vi "Camera_Crop_X_Axis_2.0.vi"(9 "Detect Movement":bool, 10 "Camera":T5, 11 "Data":T1={"Camera 1"={"Camera1"="", "Cam 1"=FALSE, "CAM1 Model"=enum."a2A5328-15ucBAS", "Cam1 ID"=0}, "Camera 2"={"Camera2"="", "Cam 2"=FALSE, "CAM2 Model"=enum."a2A5328-15ucBAS", "Cam2 ID"=0}, "Image"={"Camera1_Img"=refnum, "Camera2_Img"=refnum, "Img1_Orig_Disp"=refnum, "Img2_Orig_Disp"=refnum, "Img1_Orig_RGB"=refnum, "Img2_Orig_RGB"=refnum, "Blue_Plane_Extract"=refnum, "Subtracted_Plane"=refnum, "Img1_Binary"=refnum, "Img2_Binary"=refnum, "Crop_Mask"=refnum, "Img1_Save"=refnum, "Img2_Save"=refnum, "Img1_Cali_Full"=refnum, "Img2_Cali_Full"=refnum, "Img1_Cali_Detect"=refnum, "Img2_Cali_Detect"=refnum}, "Ques"={"Cam 1 queue"=refnum, "Cam 2 queue"=refnum, "Cam 1 - save queue"=refnum, "Cam 2 - save queue"=refnum, "Image Process Queue Size"=500, "Image Save Queue Size"=500, "Overload threshold"=500, "Max large object threshold"=0}, "Arduino SRS"={"Pinch-valve"="", "Actuator"=FALSE, "Open(T)/Close(F)"=FALSE, "Arduino Uno"=""}, "Pump"={"Port"="", "Connection"=FALSE, "Flush Size"=0, "Command"="", "Pump Size"=enum."None", "Pump"="", "Ready"=FALSE}, "Camera settings"={"Detection settings"={"Sample size threshold"=500, "Detection Region %"=30.0, "Timeout Sample"=200}, "Lens/camera settings"={"Aperture"=enum."Item 0", "Legacy Cam Attributes"=FALSE, "Max Framerate"=100, "Exposure Time"=1000.0, "Framerate"=15}, "Crop settings"={"Cam1"={"Rectangle 1"={"Left"=0, "Top"=0, "Right"=0, "Bottom"=0, "Rotation"=0.0}, "Camera Orientation 1"="", "Pixel to mm 1"=0.0}, "Cam2"={"Rectangle 2"={"Left"=0, "Top"=0, "Right"=0, "Bottom"=0, "Rotation"=0.0}, "Camera Orientation 2"="", "Pixel to mm 2"=0.0}}}, "Arduino ISS"={"Mega F3"="", "Phase3"=FALSE, "Barcode"="", "Sorting sys."=FALSE, "Initial size"=0.0, "Size Interval"=0.0, "Mun. of containers"=0.0, "Container nr."=0.0, "Arduino Mega"=""}, "Img_Capt"=FALSE, "Empty_Refill"=FALSE, "I don't think is in use"={"Light intensity"=100}, "Extended setup"={"Location"="Station", "Latitude"="Station", "Longitude"="Station", "Determiner"="Station", "Sex"="Station", "Station"="", "Collection date"=""}, "Main interface"={"Sample Name"="Test Sample", "Operator"="JFR", "Species Name"="", "Other Notes"=""}, "Tap1"=0, "SystemVersion"=0, "System Serial"="", "Exit"=FALSE, "Kuvette Full"=FALSE, "Core JKI"={"Current VI Reference"=refnum, "Close Panel on Exit?"=FALSE}, "Calibration"={"Calibration 1"=path "C:/Users/au540322/Desktop/IHS_Project/images/Debris/Debris_0/Debris_0_2019_06_01-23-32-49-686.PNG", "Calibration 2"=path "C:/Users/au540322/Desktop/IHS_Project/images/Debris/Debris_0/Debris_0_2019_06_01-23-32-49-686.PNG", "Detect 1"=path "C:/Users/au540322/Desktop/IHS_Project/images/Debris/Debris_0/Debris_0_2019_06_01-23-32-49-686.PNG", "Detect 2"=path "C:/Users/au540322/Desktop/IHS_Project/images/Debris/Debris_0/Debris_0_2019_06_01-23-32-49-686.PNG"}, "Auto Flush"=FALSE} {"SystemVersion" items=["Standard", "XL"]; "Tap1" items=["Session Data", "Extended Setup", "Buffer", "Camera", "Dispenser", "Stats", "Connections"]; "I don't think is in use"."Light intensity" scale=0.0..100.0; "Camera settings"."Crop settings"."Cam2"."Rectangle 2"."Rotation" format="%.2f"; "Camera settings"."Crop settings"."Cam2"."Rectangle 2"."Left" scale=0.0..1024.0; "Camera settings"."Crop settings"."Cam2"."Rectangle 2"."Right" scale=0.0..1024.0; "Camera settings"."Crop settings"."Cam1"."Rectangle 1"."Rotation" format="%.2f"; "Camera settings"."Crop settings"."Cam1"."Rectangle 1"."Left" scale=0.0..1024.0; "Camera settings"."Crop settings"."Cam1"."Rectangle 1"."Right" scale=0.0..1024.0; "Camera settings"."Lens/camera settings"."Framerate" min=1; "Camera settings"."Lens/camera settings"."Max Framerate" min=1; "Camera settings"."Detection settings"."Sample size threshold" min=1; "Pump"."Flush Size" min=0 max=6000 step=100; "Ques"."Overload threshold" min=1; "Ques"."Image Save Queue Size" min=1; "Ques"."Image Process Queue Size" min=1}) -> (1 "Width":i64, 3 "OffsetX":i64)   [LabVIEW 2024]
uses:
  Camera_ID.ctl
  controls/Data_JKI.ctl
  <vilib>/userDefined/High Color/IMAQdx.ctl
  <vilib>/vision/Image Controls.llb/IMAQ Image.ctl
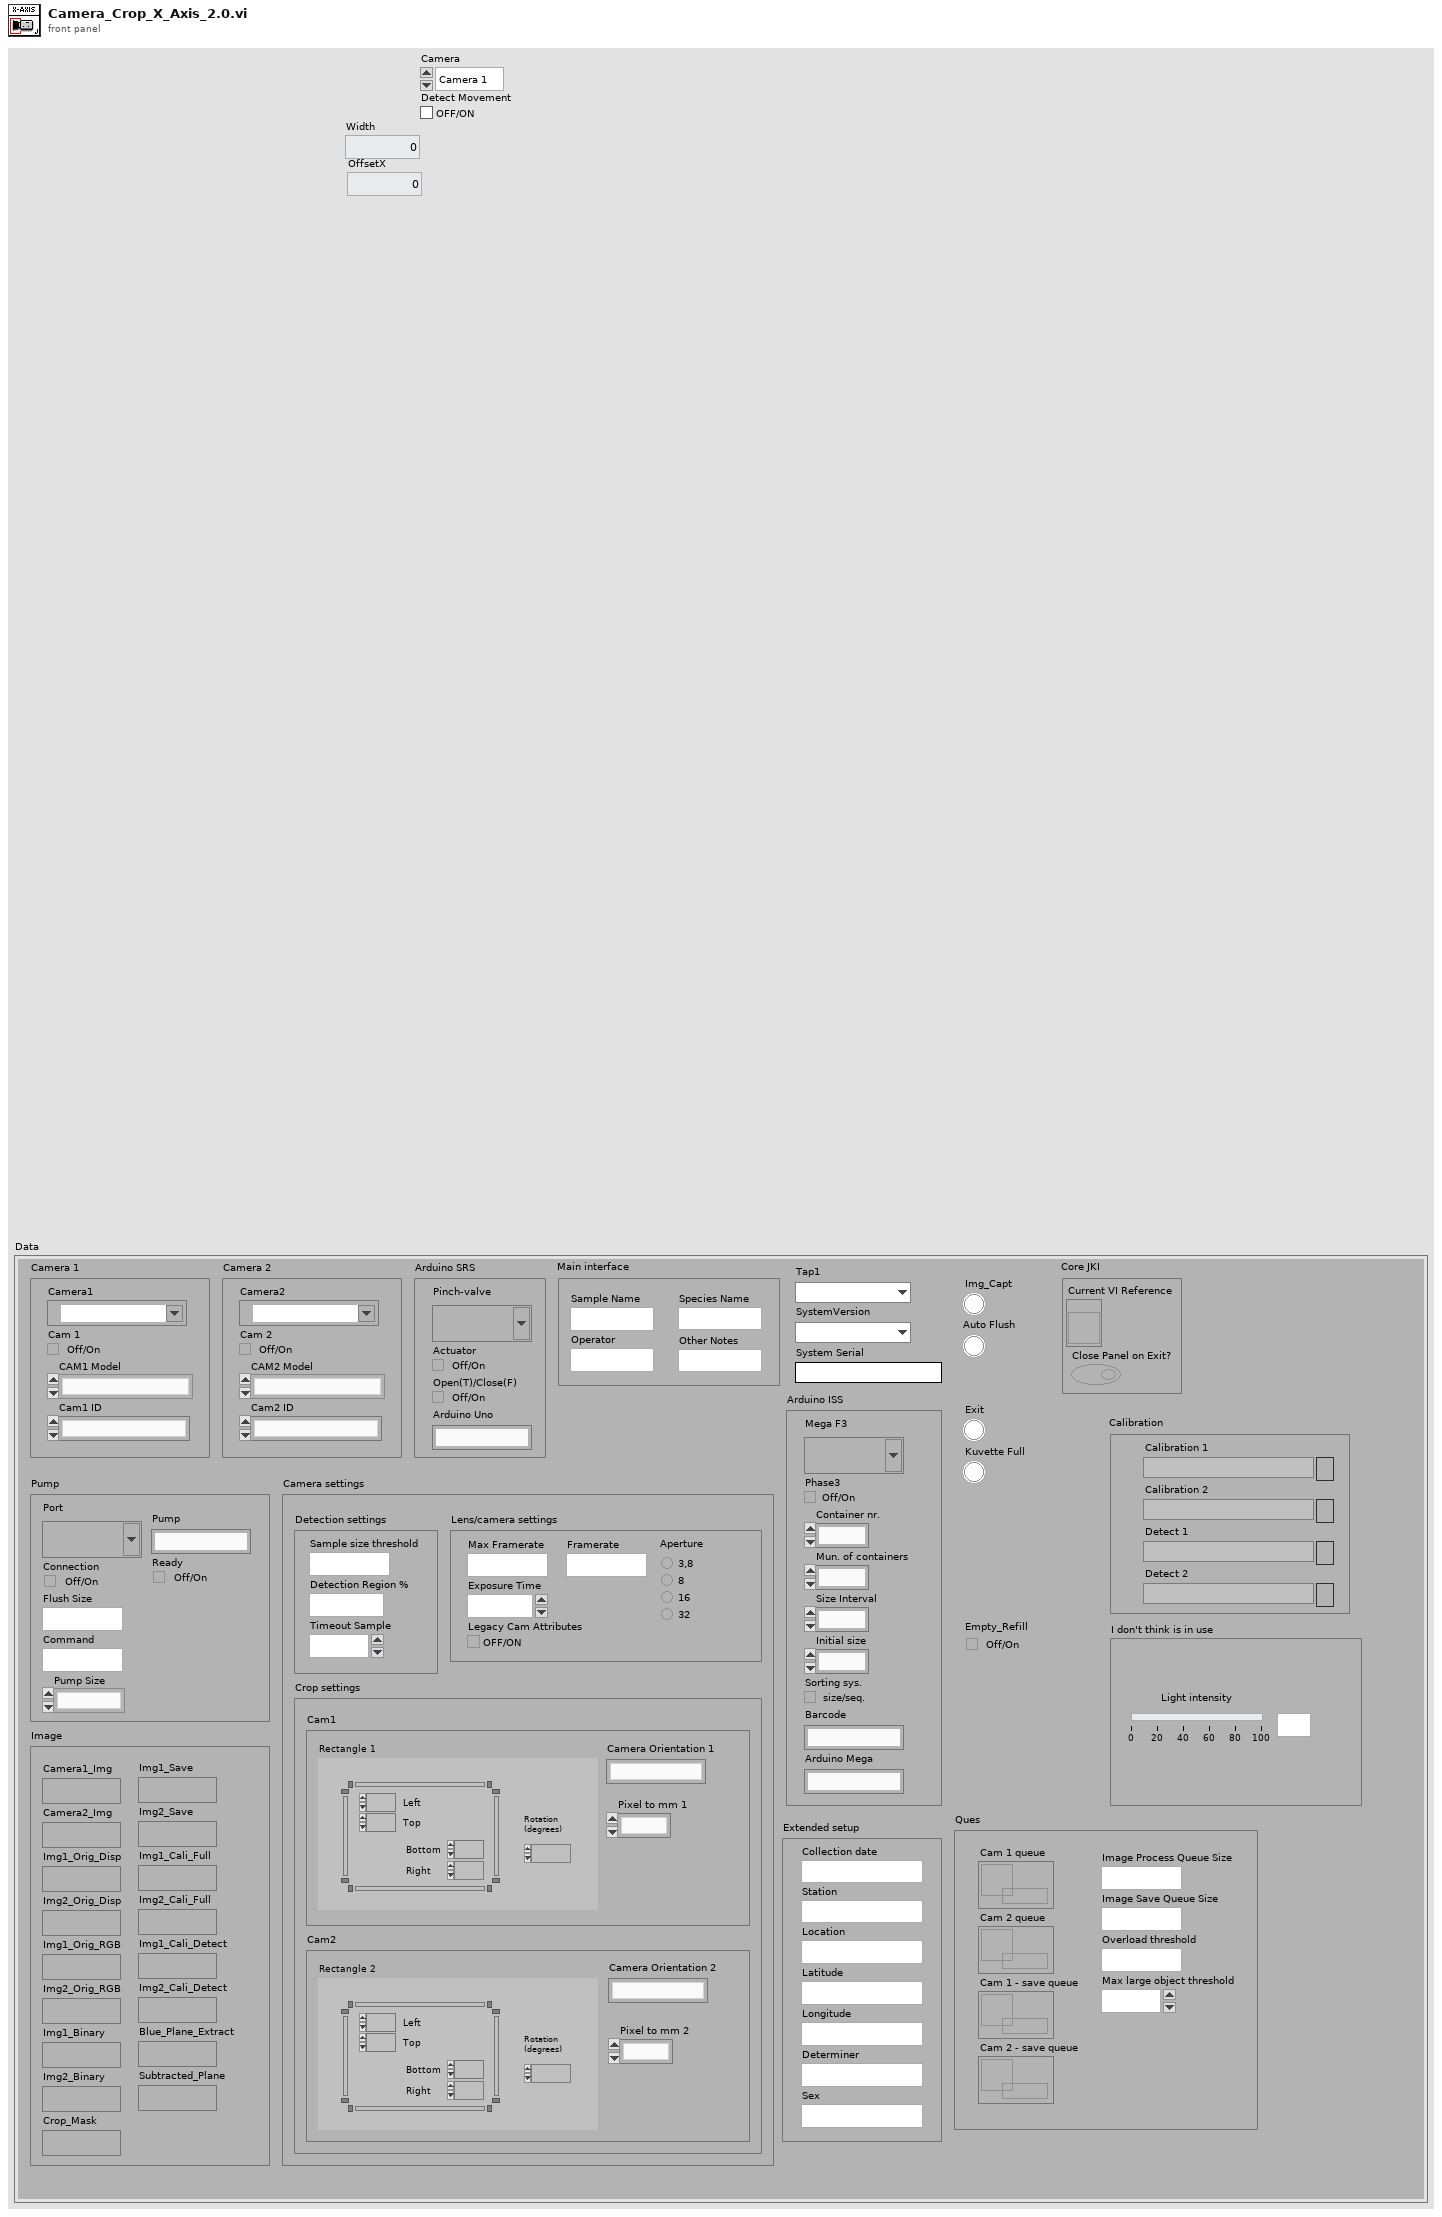
[diagram p1: front panel]
types:
  T1 = typedef "Data_JKI.ctl" = cluster{"Camera 1":cluster{"Camera1":T2, "Cam 1":bool, "CAM1 Model":enum16{"a2A5328-15ucBAS", "acA1920-155uc"}, "Cam1 ID":i32}, "Camera 2":cluster{"Camera2":T2, "Cam 2":bool, "CAM2 Model":enum16{"a2A5328-15ucBAS", "acA1920-155uc"}, "Cam2 ID":i32}, "Image":cluster{"Camera1_Img":T3, "Camera2_Img":T3, "Img1_Orig_Disp":T3, "Img2_Orig_Disp":T3, "Img1_Orig_RGB":T3, "Img2_Orig_RGB":T3, "Blue_Plane_Extract":T3, "Subtracted_Plane":T3, "Img1_Binary":T3, "Img2_Binary":T3, "Crop_Mask":T3, "Img1_Save":T3, "Img2_Save":T3, "Img1_Cali_Full":T3, "Img2_Cali_Full":T3, "Img1_Cali_Detect":T3, "Img2_Cali_Detect":T3}, "Ques":cluster{"Cam 1 queue":refnum<queue>, "Cam 2 queue":refnum<queue>, "Cam 1 - save queue":refnum<queue>, "Cam 2 - save queue":refnum<queue>, "Image Process Queue Size":i32, "Image Save Queue Size":i32, "Overload threshold":i32, "Max large object threshold":i32}, "Arduino SRS":cluster{"Pinch-valve":refnum<visa-resource-name>, "Actuator":bool, "Open(T)/Close(F)":bool, "Arduino Uno":string}, "Pump":cluster{"Port":refnum<visa-resource-name>, "Connection":bool, "Flush Size":i32, "Command":string, "Pump Size":enum16{"None", "Small", "Large"}, "Pump":string, "Ready":bool}, "Camera settings":cluster{"Detection settings":cluster{"Sample size threshold":i32, "Detection Region %":dbl, "Timeout Sample":i32}, "Lens/camera settings":cluster{"Aperture":enum32{"Item 0", "Item 1", "Item 2", "Item 3"}, "Legacy Cam Attributes":bool, "Max Framerate":i32, "Exposure Time":dbl, "Framerate":i32}, "Crop settings":cluster{"Cam1":cluster{"Rectangle 1":T4, "Camera Orientation 1":string, "Pixel to mm 1":dbl}, "Cam2":cluster{"Rectangle 2":T4, "Camera Orientation 2":string, "Pixel to mm 2":dbl}}}, "Arduino ISS":cluster{"Mega F3":refnum<visa-resource-name>, "Phase3":bool, "Barcode":string, "Sorting sys.":bool, "Initial size":dbl, "Size Interval":dbl, "Mun. of containers":dbl, "Container nr.":dbl, "Arduino Mega":string}, "Img_Capt":bool, "Empty_Refill":bool, "I don't think is in use":cluster{"Light intensity":i32}, "Extended setup":cluster{"Location":string, "Latitude":string, "Longitude":string, "Determiner":string, "Sex":string, "Station":string, "Collection date":string}, "Main interface":cluster{"Sample Name":string, "Operator":string, "Species Name":string, "Other Notes":string}, "Tap1":u16, "SystemVersion":u16, "System Serial":string, "Exit":bool, "Kuvette Full":bool, "Core JKI":cluster{"Current VI Reference":refnum<vi>, "Close Panel on Exit?":bool}, "Calibration":cluster{"Calibration 1":path, "Calibration 2":path, "Detect 1":path, "Detect 2":path}, "Auto Flush":bool}
  T2 = typedef "IMAQdx.ctl" = refnum<k21>
  T3 = typedef "IMAQ Image.ctl" = refnum<image>
  T4 = typedef "IMAQ Rectangle" = cluster{"Left":i32, "Top":i32, "Right":i32, "Bottom":i32, "Rotation":dbl}
  T5 = typedef "Camera_ID.ctl" = enum16{"Camera 1", "Camera 2"}
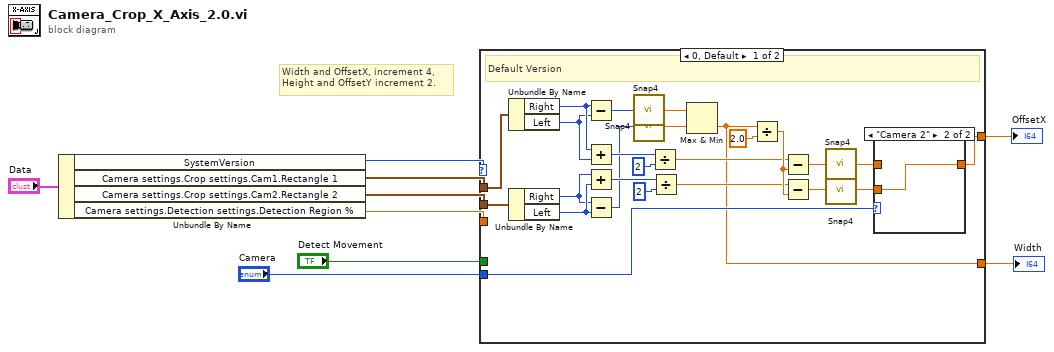
[diagram p0: block diagram]
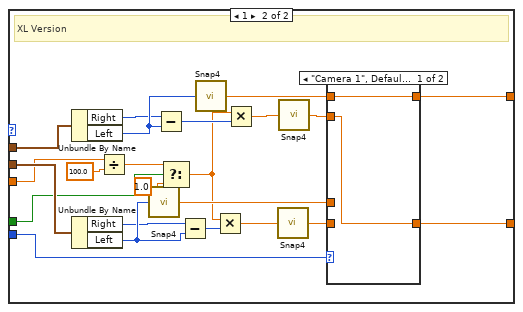
[diagram p3: hidden frame]
diagram:
  # "Width and OffsetX, increment 4,\nHeight and OffsetY increment 2."
  n1 = Unbundle By Name("Data") -> ("SystemVersion"=w6:u16, "Camera settings.Crop settings.Cam1.Rectangle 1"=w8:T4, "Camera settings.Crop settings.Cam2.Rectangle 2"=w9:T4, "Camera settings.Detection settings.Detection Region %"=w5:dbl)
  n2 = case shown="0, Default" w6 {
    tunnel: w9 -> [w30 w53]
    tunnel: w8 -> [w24 w54]
    tunnel: "Camera" -> [w22 w50]
    tunnel: [w14 w48] -> w2
    tunnel: [w19 w49] -> w3
    tunnel: w5 -> [_ w52]
    tunnel: "Detect Movement" -> [_ w51]
    frame 0, Default {
      # "Default Version"
      n3 = Unbundle By Name(w24) -> ("Right"=w16:i32, "Left"=w15:i32)
      n4 = Unbundle By Name(w30) -> ("Right"=w17:i32, "Left"=w18:i32)
      n5 = Subtract(x=w16, y=w15) -> (x-y=w10:i32)
      n6 = Add(x=w16, y=w15) -> (x+y=w25:i32)
      n7 = Add(x=w17, y=w18) -> (x+y=w28:i32)
      n8 = Subtract(x=w17, y=w18) -> (x-y=w13:i32)
      n9 = call "Snap4.vi"("x"=w10) -> ("x out"=w11:dbl)
      n10 = call "Snap4.vi"("x"=w13) -> ("x out"=w12:dbl)
      n11 = Divide(x=w25, y=2) -> (x/y=w27:dbl)
      n12 = Divide(x=w28, y=2) -> (x/y=w31:dbl)
      n13 = Max & Min(x=w11, y=w12) -> (min(x,y)=w14:dbl)  [unwired: 1 out]
      n14 = Divide(x=w14, y=2.0) -> (x/y=w32:dbl)
      n15 = Subtract(x=w27, y=w32) -> (x-y=w33:dbl)
      n16 = Subtract(x=w31, y=w32) -> (x-y=w34:dbl)
      n17 = call "Snap4.vi"("x"=w33) -> ("x out"=w21:dbl)
      n18 = call "Snap4.vi"("x"=w34) -> ("x out"=w20:dbl)
      n19 = case shown="\"Camera 2\"" w22 {
        tunnel: w21 -> [w35 _]
        tunnel: [w35 w36] -> w19
        tunnel: w20 -> [_ w36]
        frame "Camera 1", Default {
        }
        frame "Camera 2" {
        }
      }
    }
    frame 1 {
      # "XL Version"
      n20 = Unbundle By Name(w54) -> ("Right"=w40:i32, "Left"=w47:i32)
      n21 = Unbundle By Name(w53) -> ("Right"=w41:i32, "Left"=w46:i32)
      n22 = Divide(x=w52, y=100.0 ("x")) -> (x/y=w58:dbl)
      n23 = call "Snap4.vi"("x"=w46) -> ("x out"=w56:dbl)
      n24 = Subtract(x=w40, y=w47) -> (x-y=w45:i32)
      n25 = Select(t=w58, s=w51, f=1.0 ("t")) -> (s? t:f=w37:dbl)
      n26 = Subtract(x=w41, y=w46) -> (x-y=w43:i32)
      n27 = call "Snap4.vi"("x"=w47) -> ("x out"=w55:dbl)
      n28 = Multiply(x=w37, y=w43) -> (x*y=w38:dbl)
      n29 = Multiply(x=w37, y=w45) -> (x*y=w39:dbl)
      n30 = call "Snap4.vi"("x"=w38) -> ("x out"=w42:dbl)
      n31 = call "Snap4.vi"("x"=w39) -> ("x out"=w44:dbl)
      n32 = case shown="\"Camera 1\", Default" w50 {
        tunnel: w56 -> [_ w63]
        tunnel: [w61 w63] -> w49
        tunnel: w44 -> [w60 _]
        tunnel: [w60 w62] -> w48
        tunnel: w55 -> [w61 _]
        tunnel: w42 -> [_ w62]
        frame "Camera 1", Default {
        }
        frame "Camera 2" {
        }
      }
    }
  }
  "Width" <- w2
  "OffsetX" <- w3
